vi "6_position_bandwidth_main.vi"() -> ()   [LabVIEW 2019]
uses:
  Shared VIs/ENPID/PID_Settings.ctl
  Shared VIs/ENPID/Gains.ctl
  Shared VIs/ENPID/NonLinearGainParams.ctl
  Shared VIs/ENPID/NonLinearGain.ctl
  Shared VIs/ENPID/DPartVariable.ctl
  Shared VIs/ENPID/VelocityEstimate.ctl
  Shared VIs/ENPID/OutputRange.ctl
  Shared VIs/TypeDef_TDMS_States.ctl
  <vilib>/myRIO/Common/Instrument Driver Framework/myRIO v1.0/Encoder/typedefs/Encoder Signal Mode.ctl
  Shared VIs/ModelSpecific/ETHMikeModel.ctl
  Shared VIs/ModelSpecific/ReadOnlyGlobalActions.ctl
  <vilib>/myRIO/Instrument Drivers/Onboard IO/AO/typedefs/AO Reference.ctl
  <vilib>/myRIO/Common/Instrument Driver Framework/Utilities/typedefs/myRIO Generic Hardware Reference.ctl
  <vilib>/myRIO/Common/Instrument Driver Framework/Utilities/typedefs/Hardware Version Enum.ctl
  <vilib>/myRIO/Common/Instrument Driver Framework/Utilities/typedefs/myRIO v1.0 Reference.ctl
  <vilib>/myRIO/Common/Instrument Driver Framework/Utilities/typedefs/Generic FPGA Reference.ctl
  <vilib>/myRIO/Common/Instrument Driver Framework/myRIO v1.0/AO/typedefs/AO Channels List.ctl
  <vilib>/myRIO/Common/Instrument Driver Framework/myRIO v1.0/AO/typedefs/AO Channels Enum.ctl
  <vilib>/myRIO/Common/Instrument Driver Framework/Utilities/typedefs/Analog Scaling Constants List.ctl
  <vilib>/myRIO/Common/Instrument Driver Framework/Utilities/typedefs/Analog Scaling Constants.ctl
  <vilib>/userDefined/High Color/nirio_resource_hc.ctl
  <vilib>/myRIO/Instrument Drivers/Onboard IO/AI/typedefs/AI Reference.ctl
  <vilib>/myRIO/Common/Instrument Driver Framework/myRIO v1.0/AI/typedefs/AI Channels List.ctl
  <vilib>/myRIO/Common/Instrument Driver Framework/myRIO v1.0/AI/typedefs/AI Channels Enum.ctl
  <vilib>/Platform/TimedLoop/XDataNode/timing_clust.ctl
  <vilib>/Platform/TimedLoop/XDataNode/nitl_modes.ctl
  <vilib>/Platform/TimedLoop/XDataNode/wakeup.ctl
  <vilib>/Analysis/3filter.llb/Filter Passband Type.ctl
  <vilib>/myRIO/Common/Instrument Driver Framework/myRIO v1.0/AO/vis/myRIO v1.1 Open AO.vi
  <vilib>/myRIO/Common/Instrument Driver Framework/myRIO v1.0/AI/vis/myRIO v1.1 Open AI.vi
  <vilib>/myRIO/Common/Instrument Driver Framework/Utilities/vis/Validate Channels.vi
  <vilib>/myRIO/Common/Instrument Driver Framework/myRIO v1.0/AO/vis/myRIO v1.0 Reserve AO.vi
  <vilib>/myRIO/Common/Instrument Driver Framework/myRIO v1.0/AI/vis/myRIO v1.0 Reserve AI.vi
  <vilib>/myRIO/Common/Instrument Driver Framework/myRIO v1.0/AO/vis/myRIO v1.0 Close AO.vi
  <vilib>/myRIO/Common/Instrument Driver Framework/myRIO v1.0/AI/vis/myRIO v1.0 Close AI.vi
  <vilib>/myRIO/Common/Instrument Driver Framework/myRIO v1.0/Encoder/vis/myRIO v1.0 Close Encoder.vi
  <vilib>/myRIO/Common/Instrument Driver Framework/myRIO v1.0/AO/vis/myRIO v1.0 Build MUX Configuration AO.vi
  <vilib>/myRIO/Common/Instrument Driver Framework/myRIO v1.0/Resource Manager/vis/myRIO v1.0 Reserve Channel List.vi
  <vilib>/myRIO/Common/Instrument Driver Framework/myRIO v1.0/AI/vis/myRIO v1.0 Build MUX Configuration AI.vi
  <vilib>/myRIO/Common/Instrument Driver Framework/myRIO v1.0/AO/vis/myRIO v1.0 Unreserve AO.vi
  <vilib>/myRIO/Common/Instrument Driver Framework/myRIO v1.0/AI/vis/myRIO v1.0 Unreserve AI.vi
  <vilib>/myRIO/Common/Instrument Driver Framework/myRIO v1.0/Encoder/vis/myRIO v1.0 Unreserve Encoder.vi
  <vilib>/myRIO/Common/Instrument Driver Framework/myRIO v1.0/Resource Manager/vis/myRIO v1.0 Reserve Channel.vi
  <vilib>/myRIO/Common/Instrument Driver Framework/myRIO v1.0/Resource Manager/vis/myRIO v1.0 Unreserve Channel.vi
  <vilib>/myRIO/Common/Instrument Driver Framework/myRIO v1.0/Resource Manager/vis/myRIO v1.0 Unreserve Channel List.vi
  <vilib>/myRIO/Common/Instrument Driver Framework/myRIO v1.0/Encoder/vis/myRIO v1.0 Build MUX Configuration Encoder.vi
  <vilib>/myRIO/Common/Instrument Driver Framework/myRIO v1.0/Resource Manager/vis/myRIO v1.0 Build Mutex Name.vi
  <vilib>/myRIO/Common/Instrument Driver Framework/myRIO v1.0/Resource Manager/vis/myRIO v1.0 Create Configuration List.vi
  <vilib>/Utility/VariantDataType/GetNumericInfo.vi
  <vilib>/Utility/error.llb/Error Cluster From Error Code.vi
  <vilib>/myRIO/Common/Instrument Driver Framework/myRIO v1.0/myRIO v1.1 Open.vi
  <vilib>/myRIO/Common/Instrument Driver Framework/myRIO v1.0/AO/vis/myRIO v1.0 Get Scaling Constants AO.vi
  <vilib>/myRIO/Common/Instrument Driver Framework/Utilities/vis/IO Manager.vi
  <vilib>/myRIO/Common/Instrument Driver Framework/Utilities/vis/Configuration Manager.vi
  <vilib>/myRIO/Common/Instrument Driver Framework/myRIO v1.0/myRIO v1.0 Close.vi
  <vilib>/myRIO/Common/Instrument Driver Framework/myRIO v1.0/AO/vis/myRIO v1.0 Write AO.vi
  <vilib>/myRIO/Common/Instrument Driver Framework/myRIO v1.0/AI/vis/myRIO v1.0 Get Scaling Constants AI.vi
  <vilib>/myRIO/Common/Instrument Driver Framework/myRIO v1.0/Encoder/vis/myRIO v1.0 Read Encoder.vi
  <vilib>/myRIO/Common/Instrument Driver Framework/myRIO v1.0/AI/vis/myRIO v1.0 Read AI.vi
  <vilib>/myRIO/Common/Instrument Driver Framework/myRIO v1.0/Encoder/vis/myRIO v1.0 Enable Encoder.vi
  <vilib>/myRIO/Common/Instrument Driver Framework/myRIO v1.0/Encoder/vis/myRIO v1.0 Shutdown Encoder.vi
  <vilib>/myRIO/Common/Instrument Driver Framework/myRIO v1.0/Resource Manager/vis/myRIO v1.0 Configure IO.vi
  <vilib>/myRIO/Instrument Drivers/Onboard IO/AO/vis/myRIO AO Open.xnode
  <vilib>/myRIO/Instrument Drivers/Onboard IO/AI/vis/myRIO AI Open.xnode
  <vilib>/platform/TimedLoop/XDataNode/XDataNode.xnode
  <vilib>/myRIO/Instrument Drivers/Onboard IO/AO/AO.lvlib
  <vilib>/myRIO/Instrument Drivers/Onboard IO/Encoder/Encoder.lvlib
  <vilib>/myRIO/Instrument Drivers/Onboard IO/AI/AI.lvlib
  <vilib>/Platform/TimedLoop/XDataNode/XDNodeRunTimeDep.lvlib
  <vilib>/Analysis/NI_AALBase.lvlib
  <vilib>/ptbypt/NI_PtbyPt.lvlib
  <vilib>/addons/control/pid/NI_PID_pid.lvlib
panel:
  out "Velocity [deg/s]":dbl(graph)
  out "TDMS States":T1
  in  "TDMS Storage File Input":string
  in  "PID Settings":T2={"Gains"={"K(e)"=0.0, "Kp"=0.800000011920929, "Ki"=0.0, "Kd"=0.003000000026077032}, "Non-linear gain"={"Non-linear gain P"=enum."off", "Non-linear gain I"=enum."off", "Non-linear gain D"=enum."off"}, "D-Part variable"=enum."process variable", "Velocity estimate dy/dt"=enum."external", "Anti reset windup"=TRUE, "I-Part error band"=inf, "Output range"={"output high"=0.0, "output low"=0.0}}
  in  "Sine Amplitude (deg)":dbl
  out "Current Setpoint [A]":dbl(graph)
  out "i":dbl
  out "Velocity Unfiltered [deg/s]":dbl
  out "Position [deg]":cluster{"Position [deg]":dbl, "setpoint":dbl}(graph)
  out "Time (s)":dbl
  out "Velocity [deg/s]":dbl
  out "Current Setpoint [A]":dbl
  out "Position Setpoint [deg]":dbl
  in  "Sine Frequency (Hz)":dbl
  in  "Cycles":dbl
  in  "run":bool
  in  "Save data?":bool
  out "Position [deg]":dbl
  in  "stop":bool
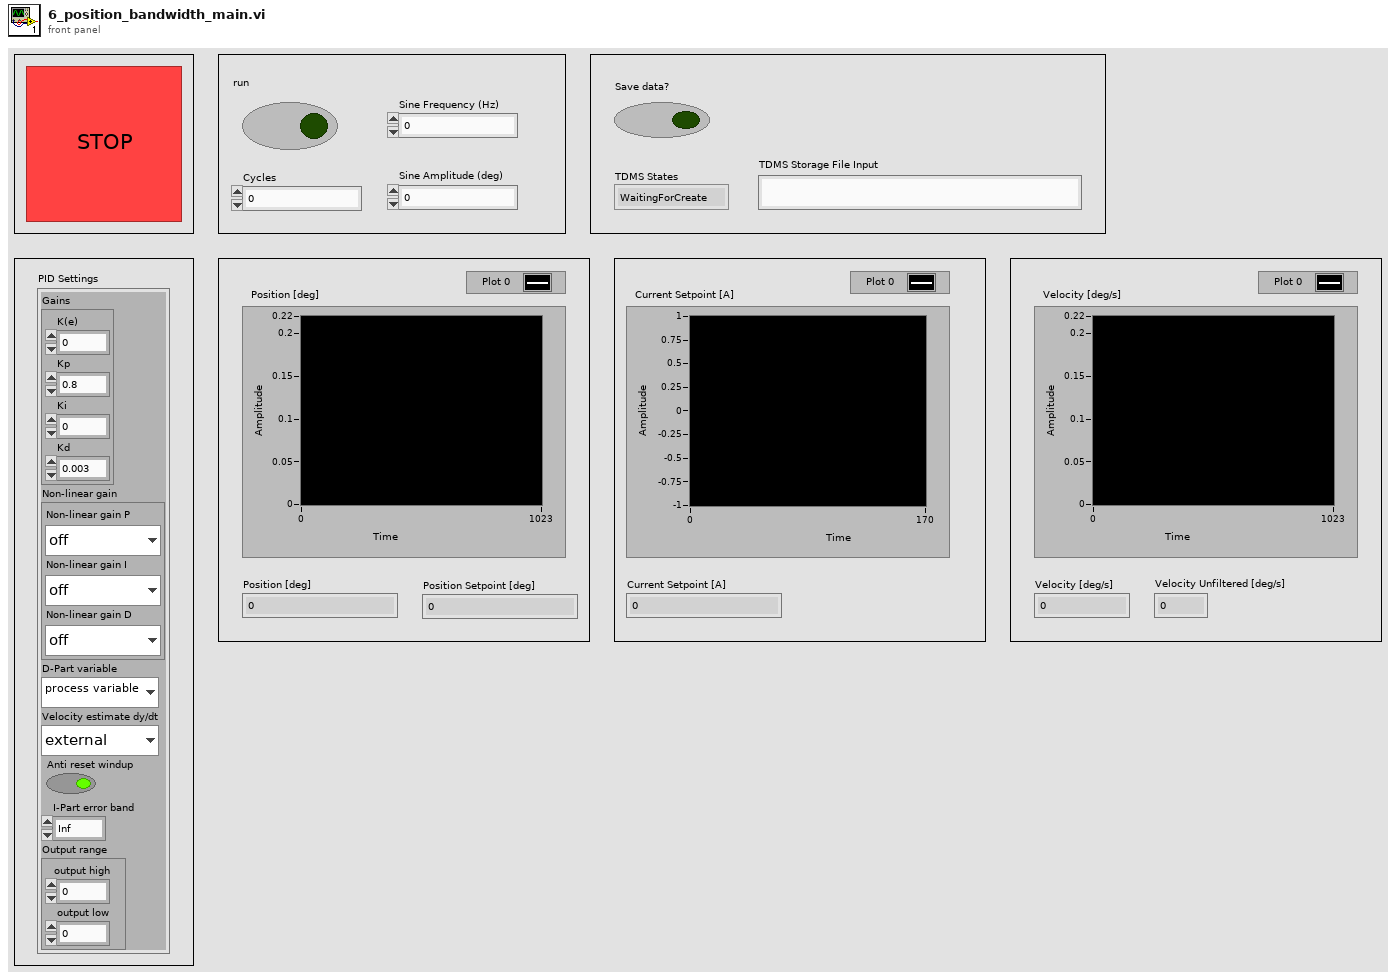
[diagram p1: front panel]
types:
  T1 = typedef "TypeDef_TDMS_States.ctl" = enum16{"WaitingForCreate", "Create", "Buffering", "Flushing", "Write", "Close"}
  T2 = typedef "PID_Settings.ctl" = cluster{"Gains":T3, "Non-linear gain":T4, "D-Part variable":T6, "Velocity estimate dy/dt":T7, "Anti reset windup":bool, "I-Part error band":dbl, "Output range":T8}
  T3 = typedef "Gains.ctl" = cluster{"K(e)":dbl, "Kp":dbl, "Ki":dbl, "Kd":dbl}
  T4 = typedef "NonLinearGainParams.ctl" = cluster{"Non-linear gain P":T5, "Non-linear gain I":T5, "Non-linear gain D":T5}
  T5 = typedef "NonLinearGain.ctl" = enum16{"exponential", "quadratic", "off"}
  T6 = typedef "DPartVariable.ctl" = enum16{"error", "process variable"}
  T7 = typedef "VelocityEstimate.ctl" = enum16{"derivative", "external"}
  T8 = typedef "OutputRange.ctl" = cluster{"output high":dbl, "output low":dbl}
  T9 = typedef "nirio_resource_hc.ctl" = tag
  T10 = typedef "Hardware Version Enum.ctl" = enum16{"Unknown", "myRIO-1900", "myRIO-1950", "roboRIO", "NI ELVIS RIO CM", "ELVIS III"}
  T11 = enum16{"open", "open or create", "create or replace", "create", "open (read-only)"}
  T12 = typedef "XDNodeRunTimeDep.lvlib/timing_clust.ctl" = cluster{"Expected End [f-1]":u64, "Actual End [f-1]":u64, "Finished Late? [f-1]":bool, "Expected End [i-1]":u64, "Actual End [i-1]":u64, "Finished Late? [i-1]":bool, "Expected Start [i]":u64, "Actual Start [i]":u64, "Expected Start [f]":u64, "Actual Start [f]":u64, "Source Name":string, "Structure Name":string, "Period":i64, "Deadline":i64, "Offset":i64, "Start":i64, "Priority":i32, "Timeout":i32, "Mode":T13, "Wakeup Reason":T14, "Error":errorcluster, "Source Type":string, "Secondary Source Type":string, "Global End Time":u64, "Global Start Time":u64, "Frame Duration":u64, "Iteration Duration":u64, "Assigned CPU":i32, "I/O Scan Engine Mode":u32}
  T13 = typedef "XDNodeRunTimeDep.lvlib/nitl_modes.ctl" = enum32{"No Change", "Process missed periods, maintain original phase", "Discard missed periods, maintain original phase", "Process missed periods, ignore original phase", "Discard missed periods, ignore original phase"}
  T14 = typedef "XDNodeRunTimeDep.lvlib/wakeup.ctl" = enum32{"Normal", "Aborted", "Asynchronous wakeup", "Timing source error", "Timed loop error", "Timeout"}
  T15 = typedef "NI_AALBase.lvlib/Filter Passband Type.ctl" = enum32{"Lowpass", "Highpass", "Bandpass", "Bandstop"}
  T16 = typedef "ReadOnlyGlobalActions.ctl" = enum16{"Initialize", "Read", "Write"}
  T17 = typedef "ETHMikeModel.ctl" = enum16{"ETH Mike #1", "ETH Mike #2", "ETH Mike #3", "ETH Mike #4", "ETH MIKE #5"}
  T18 = typedef "Encoder Signal Mode.ctl" = enum16{"Quadrature phase signal", "Step and direction signal"}
  T19 = typedef "AO.lvlib/AO Reference.ctl" = cluster{"myRIO Reference":T20, "AO Channel List":T23, "AO Scaling Constant List":T25}
  T20 = typedef "myRIO Generic Hardware Reference.ctl" = cluster{"myRIO Model":T10, "myRIO Hardware Reference":T21}
  T21 = typedef "myRIO v1.0 Reference.ctl" = cluster{"Generic FPGA Reference":T22, "Allow multiple opens":bool}
  T22 = typedef "Generic FPGA Reference.ctl" = refnum<k20>
  T23 = typedef "AO Channels List.ctl" = T24[]
  T24 = typedef "AO Channels Enum.ctl" = enum16{"Not Connected", "AudioOut/Left", "AudioOut/Right", "C/AO0", "C/AO1", "A/AO0", "A/AO1", "B/AO0", "B/AO1"}
  T25 = typedef "Analog Scaling Constants List.ctl" = T26[]
  T26 = typedef "Analog Scaling Constants.ctl" = cluster{"LSB Weight (Volts)":dbl, "Offset (Volts)":dbl, "Signed?":bool}
  T27 = typedef "Encoder.lvlib/Encoder Reference.ctl" = cluster{"myRIO Reference":T20, "Encoder Channels Enum":T28}
  T28 = typedef "Encoder Channels Enum.ctl" = enum16{"Not Connected", "C/ENC0", "C/ENC1", "A/ENC", "A/ENC0", "A/ENC1", "A/ENC2", "A/ENC3", "A/ENC4", "A/ENC5", "A/ENC6", "A/ENC7", "A/ENC8", "A/ENC9", "B/ENC", "B/ENC0", "B/ENC1", "B/ENC2", "B/ENC3", "B/ENC4", "B/ENC5", "B/ENC6", "B/ENC7", "B/ENC8", "B/ENC9", "DIO/ENC0", "DIO/ENC1", "DIO/ENC2", "DIO/ENC3", "DIO/ENC4"}
  T29 = typedef "AI.lvlib/AI Reference.ctl" = cluster{"myRIO Reference":T20, "AI Channels List":T30, "AI Scaling Constants List":T25}
  T30 = typedef "AI Channels List.ctl" = T31[]
  T31 = typedef "AI Channels Enum.ctl" = enum16{"Not Connected", "AudioIn/Left", "AudioIn/Right", "C/AI0", "C/AI1", "A/AI0", "A/AI1", "A/AI2", "A/AI3", "A/AI4", "A/AI5", "A/AI6", "A/AI7", "B/AI0", "B/AI1", "B/AI2", "B/AI3", "B/AI4", "B/AI5", "B/AI6", "B/AI7", "AI/AI0", "AI/AI1", "AI/AI2", "AI/AI3", "A/AI0 (DIFF)", "A/AI1 (DIFF)", "A/AI2 (DIFF)", "A/AI3 (DIFF)", "B/AI0 (DIFF)", "B/AI1 (DIFF)", "B/AI2 (DIFF)", "B/AI3 (DIFF)"}
  T32 = typedef "TypeDefTachometerParam.ctl" = cluster{"Offset [V]":dbl, "Gain [deg/sV]":dbl}
  T33 = cluster{"Position [deg]":dbl, "Position [deg]":dbl}
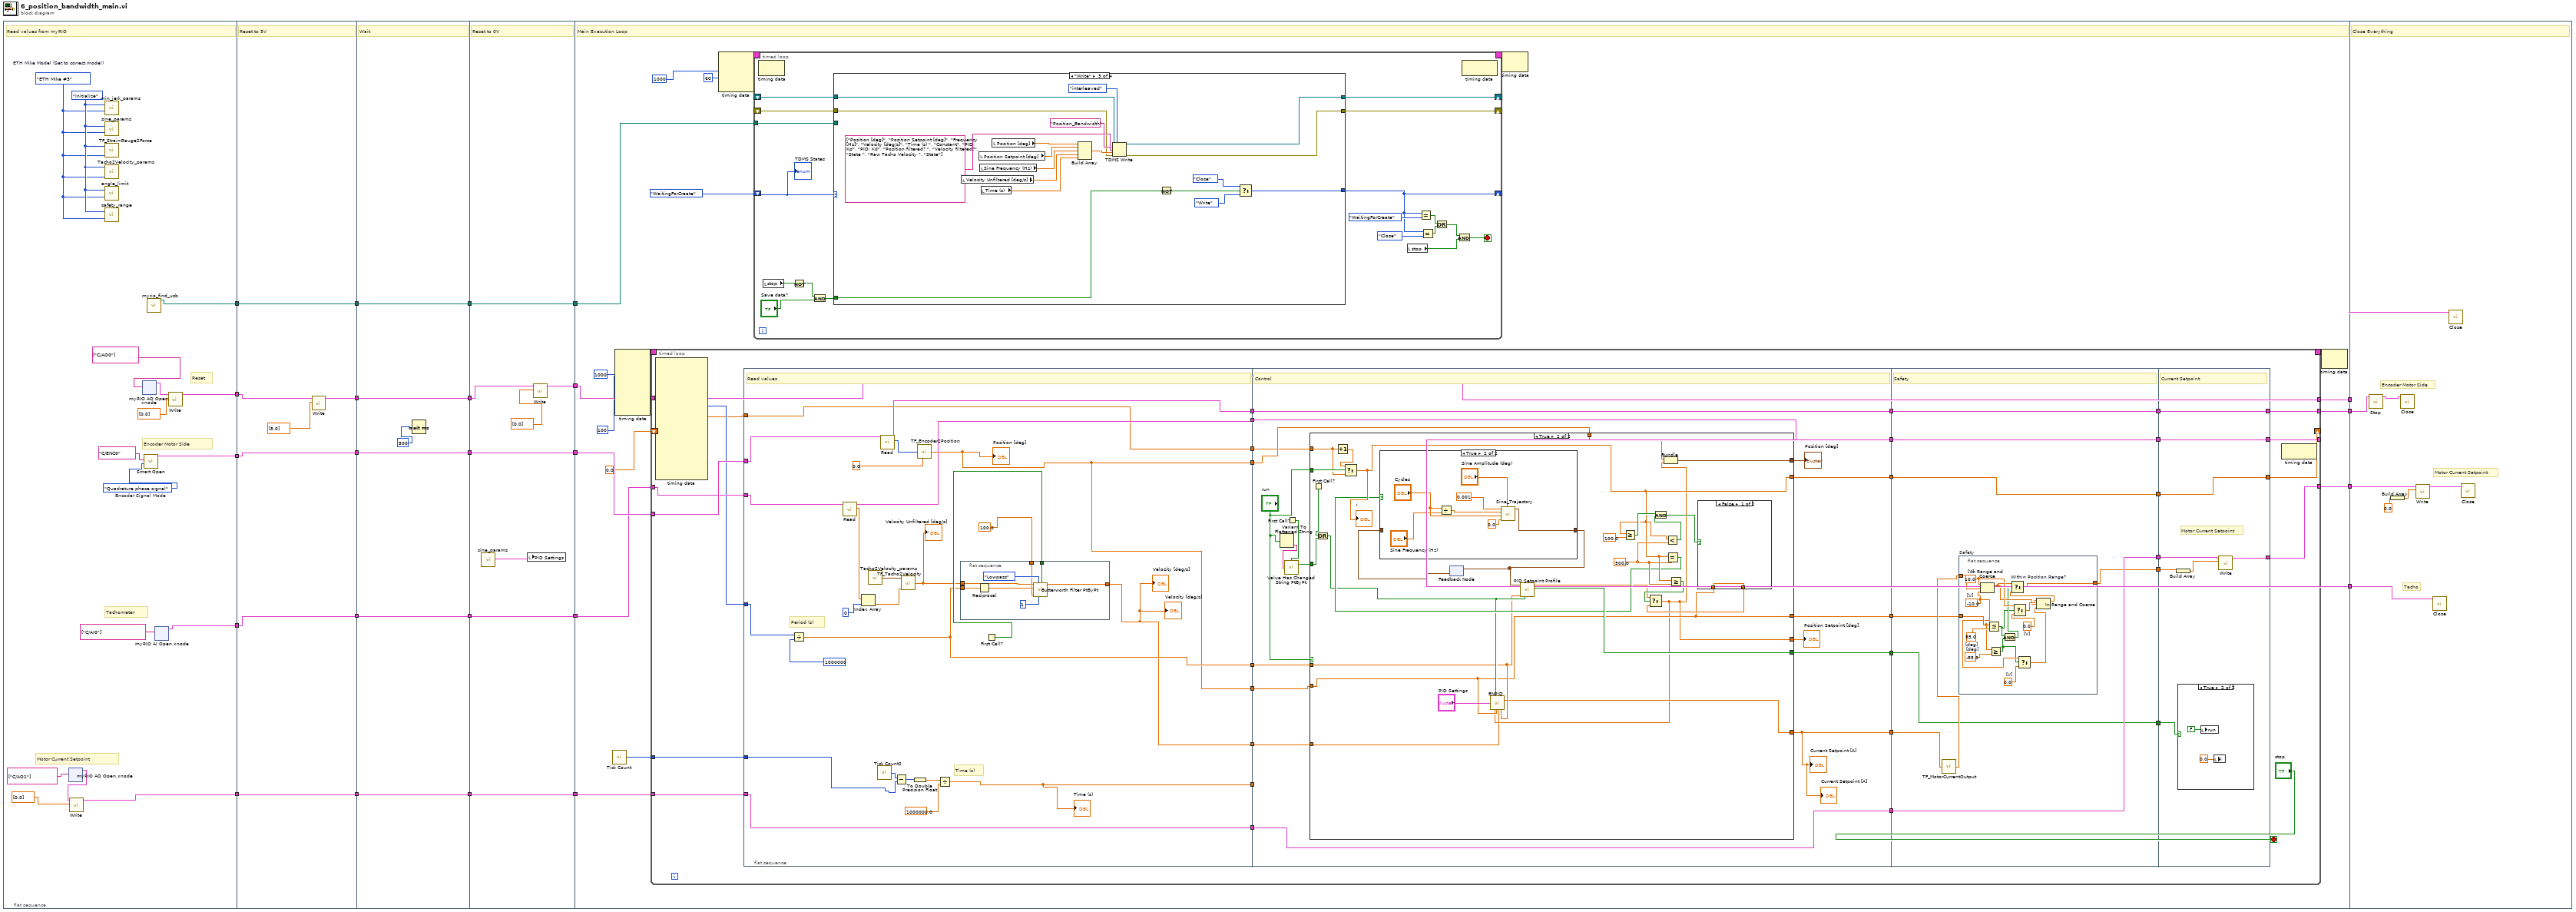
[diagram p0: block diagram]
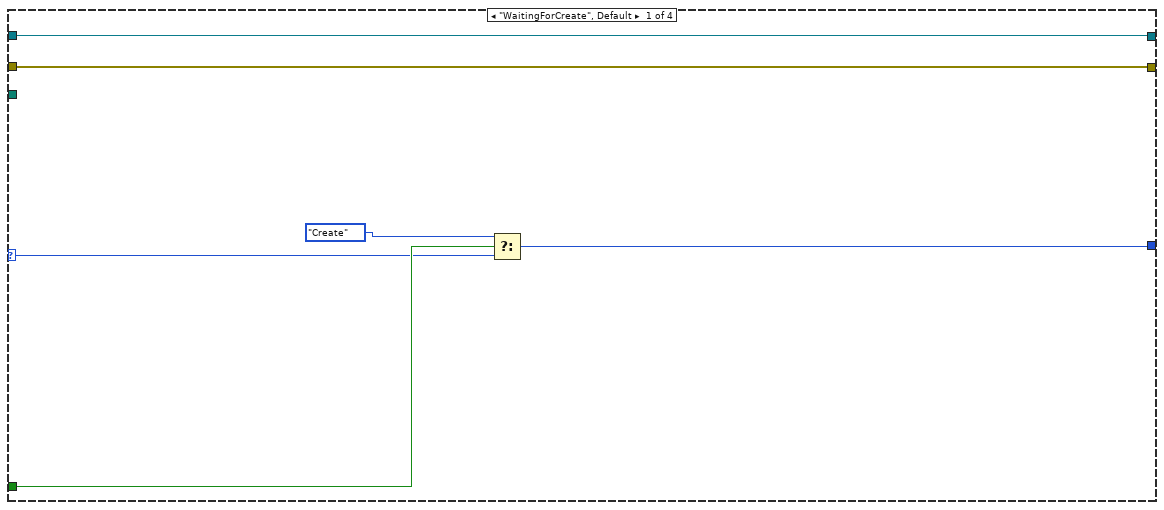
[diagram p2: hidden frame]
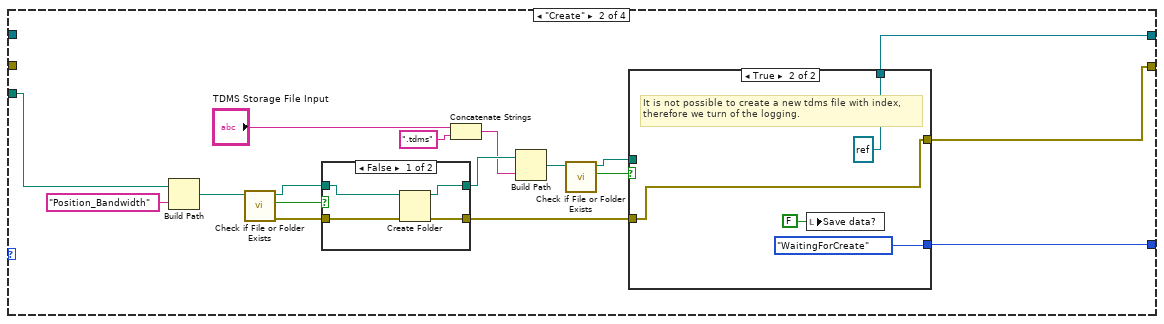
[diagram p3: hidden frame]
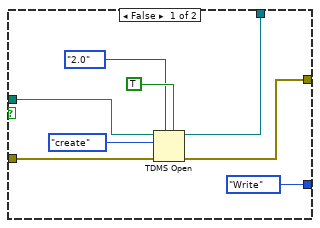
[diagram p4: hidden frame]
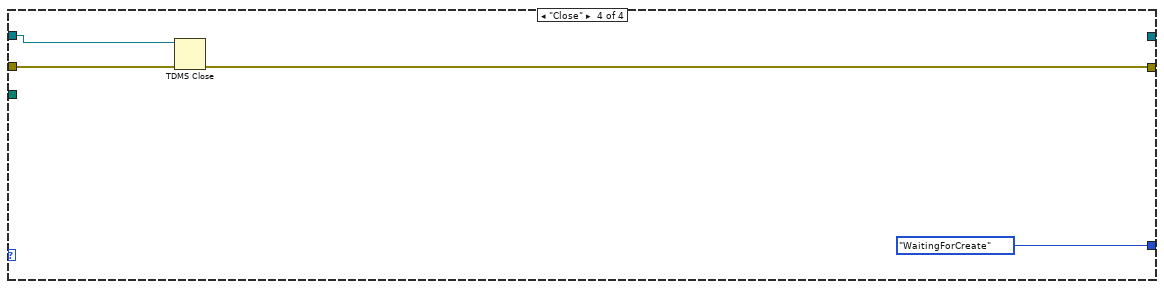
[diagram p6: hidden frame]
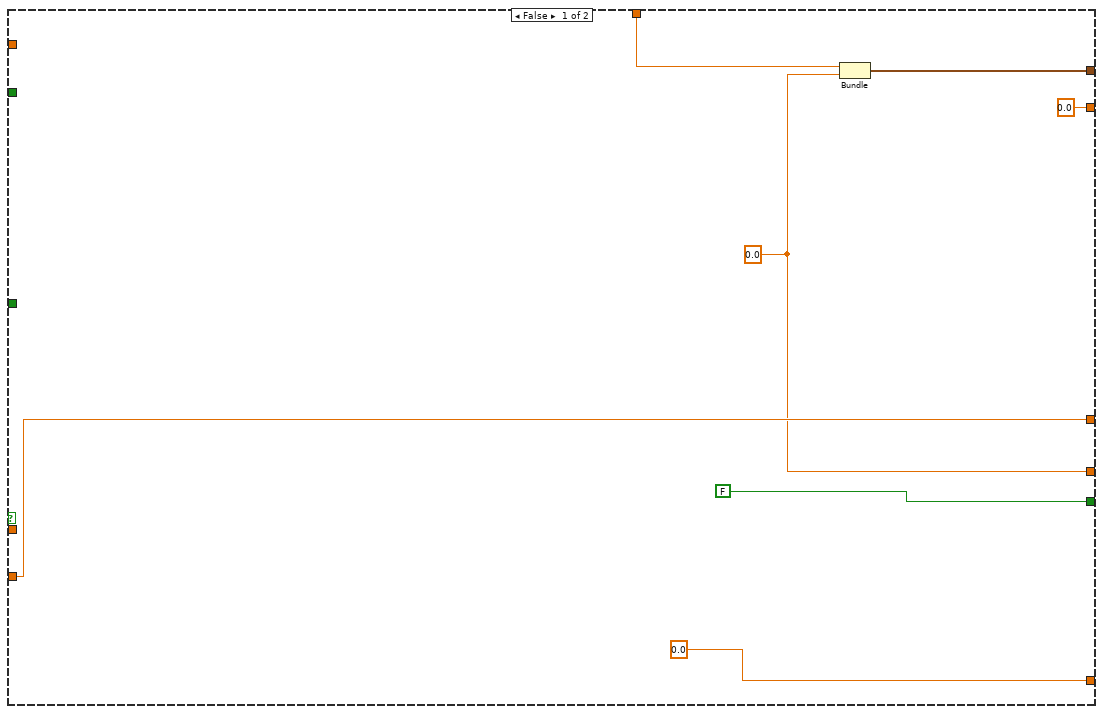
[diagram p7: hidden frame]
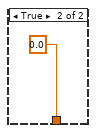
[diagram p8: hidden frame]
diagram:
  n1 = flat-sequence {
    tunnel: [w34] -> w24
    tunnel: [w33] -> w23
    tunnel: [w32] -> w22
    tunnel: [w31] -> w21
    tunnel: [w27] -> w2
    tunnel: w24 -> [w96]
    tunnel: w23 -> [w100]
    tunnel: w22 -> [w98]
    tunnel: w21 -> [w97]
    tunnel: [w99] -> w20
    tunnel: [w98] -> w15
    tunnel: [w97] -> w12
    tunnel: [w96] -> w6
    tunnel: [w95] -> w3
    tunnel: w2 -> [w95]
    tunnel: w20 -> [w106]
    tunnel: [w106] -> w19
    tunnel: [w105] -> w16
    tunnel: w15 -> [w105]
    tunnel: [w104] -> w13
    tunnel: w12 -> [w104]
    tunnel: [w103] -> w7
    tunnel: w6 -> [w103]
    tunnel: [w102] -> w4
    tunnel: w3 -> [w102]
    tunnel: w19 -> [w114]
    tunnel: [w113] -> w18
    tunnel: [w112] -> w17
    tunnel: w16 -> [w112]
    tunnel: [w111] -> w14
    tunnel: w13 -> [w111]
    tunnel: [w110] -> w8
    tunnel: w7 -> [w110]
    tunnel: [w109] -> w5
    tunnel: w4 -> [w109]
    tunnel: w18 -> [w132]
    tunnel: w17 -> [w131]
    tunnel: w14 -> [w129]
    tunnel: [w120] -> w11
    tunnel: [w130] -> w10
    tunnel: [w128] -> w9
    tunnel: w8 -> [w125]
    tunnel: w5 -> [w122]
    tunnel: [w121] -> w1
    tunnel: w11 -> [w404]
    tunnel: w10 -> [w402]
    tunnel: w9 -> [w401]
    tunnel: w1 -> [w399]
    frame #0 {
      w26 = ReadOnlyGlobalActions."Initialize" ("Action (Read)")
      w25 = ETHMikeModel."ETH Mike #3"  # ETH Mike Model (Set to correct model)
      w36 = Encoder_Signal_Mode."Quadrature phase signal"  # Encoder Signal Mode
      # "Motor Current Setpoint"
      # "Tachometer"
      # "Encoder Motor Side"
      # "Reset"
      # "Read values from myRIO"
      n2 = xnode "myRIO AO Open.xnode"("Channel Names"=tag[] ["C/AO1"]) -> ("AO Ref Out"=w29:T19)  [unwired: 2 in, 1 out]
      n3 = call <vilib>:"Write.vi"("Values"=dbl[] [0.0], "AO Ref In"=w29) -> ("AO Ref Out"=w27:T19)  [unwired: 7 in, 1 out]
      n4 = call "min_jerk_params.vi"("Action (Read)"=w26, "ETH Mike Model"=w25) -> ()  [unwired: 17 in, 1 out]
      n5 = call "sine_params.vi"("Action (Read)"=w26, "ETH Mike Model"=w25) -> ()  [unwired: 17 in, 1 out]
      n6 = call "TF_StrainGauge2Force.vi"("Action (Read)"=w26, "ETH Mike Model"=w25) -> ()  [unwired: 3 in, 1 out]
      n7 = call "Tacho2Velocity_params.vi"("Action (Read)"=w26, "ETH Mike Model"=w25) -> ()  [unwired: 3 in, 1 out]
      n8 = call "angle_limit.vi"("ETH Mike Model"=w25, "Action (Read)"=w26) -> ()  [unwired: 1 out]
      n9 = call "safety_range.vi"("ETH Mike Model"=w25, "Action (Read)"=w26) -> ()  [unwired: 1 out]
      n10 = xnode "myRIO AO Open.xnode"("Channel Names"=tag[] ["C/AO0"]) -> ("AO Ref Out"=w39:T19)  [unwired: 2 in, 1 out]
      n11 = call <vilib>:"Smart Open.vi"("Encoder Signal Mode"=w36, "Channel Name"=tag "C/ENC0") -> ("Encoder Ref Out"=w32:T27)  [unwired: 8 in, 1 out]
      n12 = call "myrio_find_usb.vi"() -> ("Largest USB Partition Path"=w34:path)  [unwired: 9 in, 2 out]
      n13 = xnode "myRIO AI Open.xnode"("Channel Names"=tag[] ["C/AI0"]) -> ("AI Ref Out"=w31:T29)  [unwired: 2 in, 1 out]
      n14 = call <vilib>:"Write.vi"("Values"=dbl[] [0.0], "AO Ref In"=w39) -> ("AO Ref Out"=w33:T19)  [unwired: 7 in, 1 out]
    }
    frame #1 {
      # "Reset to 5V"
      n15 = call <vilib>:"Write.vi"("Values"=dbl[] [5.0], "AO Ref In"=w100) -> ("AO Ref Out"=w99:T19)  [unwired: 7 in, 1 out]
    }
    frame #2 {
      # "Wait"
      n16 = Wait (ms)(milliseconds to wait=500) -> ()  [unwired: 1 out]
    }
    frame #3 {
      # "Reset to 0V"
      n17 = call "sine_params.vi"() -> ("PID Settings"=w108:T2)  [unwired: 19 in]
      n18 = local write "PID Settings"(w108) -> ()
      n19 = call <vilib>:"Write.vi"("Values"=dbl[] [0.0], "AO Ref In"=w114) -> ("AO Ref Out"=w113:T19)  [unwired: 7 in, 1 out]
    }
    frame #4 {
      # "Main Execution Loop"
      n20 = call "Tick Count"() -> ("Tick Count(uSec)"=w123:u32)
      n21 = node-c288(i64 1000 ("Period"), 100) -> (w135:T12)  [unwired: 6 in]
      n22 = timed-loop {
        timing: w135 -> [_]
        timing-out: [_] -> w134
        tunnel: [w257] -> w120
        tunnel: w132 -> [w257]
        tunnel: w131 -> [w256]
        tunnel: [w255] -> w130
        tunnel: w129 -> [w254]
        tunnel: [w253] -> w128
        tunnel: w123 -> [w244]
        tunnel: w122 -> [w237]
        tunnel: [w233] -> w121
        shift-right: [w227] -> _
        shift-left: 0.0 -> [w224]
        stop <- "stop" stop-if-true
        n23 = node-c288() -> (w252:i64)  [unwired: 1 in, 16 out]
        n24 = flat-sequence {
          tunnel: [w283] -> w251
          tunnel: [w273] -> w249
          tunnel: w252 -> [w281]
          tunnel: w254 -> [w282]
          tunnel: w256 -> [w274]
          tunnel: w244 -> [w268]
          tunnel: [w265] -> w243
          tunnel: [w267] -> w242
          tunnel: [w258] -> w241
          tunnel: [w264] -> w240
          tunnel: w237 -> [w266]
          tunnel: [w266] -> w236
          tunnel: [w264] -> w230
          tunnel: [w262] -> w228
          tunnel: w224 -> [w262]
          tunnel: w251 -> [w309]
          tunnel: [w309] -> w250
          tunnel: w249 -> [w308]
          tunnel: [w308] -> w248
          tunnel: w243 -> [_]
          tunnel: w242 -> [w307]
          tunnel: w241 -> [w303]
          tunnel: w240 -> [w302]
          tunnel: [w301] -> w239
          tunnel: w236 -> [w300]
          tunnel: [w300] -> w235
          tunnel: [w299] -> w231
          tunnel: w230 -> [w298]
          tunnel: [w294] -> w229
          tunnel: w228 -> [w297]
          tunnel: [w295] -> w225
          tunnel: w250 -> [w362]
          tunnel: w248 -> [w361]
          tunnel: [w362] -> w246
          tunnel: [w361] -> w245
          tunnel: w239 -> [w359]
          tunnel: [w354] -> w238
          tunnel: w235 -> [w358]
          tunnel: [w358] -> w234
          tunnel: [w357] -> w232
          tunnel: w231 -> [w357]
          tunnel: w229 -> [w356]
          tunnel: [w355] -> w226
          tunnel: w225 -> [w355]
          tunnel: [w385] -> w253
          tunnel: [w386] -> w255
          tunnel: w246 -> [w386]
          tunnel: w245 -> [w385]
          tunnel: w238 -> [w384]
          tunnel: [w382] -> w233
          tunnel: w234 -> [w381]
          tunnel: w232 -> [w380]
          tunnel: [w379] -> w227
          tunnel: w226 -> [w379]
          frame #0 {
            # "Time (s)"
            # "Period (s)"
            # "Read values"
            n25 = Divide(x=w281, y=1000000) -> (x/y=w267:dbl)
            n26 = call <vilib>:"Read.vi"("AI Ref In"=w282) -> ("Values"=w278:dbl[], "AI Ref Out"=w273:T29)  [unwired: 8 in, 1 out]
            n27 = Index Array(array=w278, index=0) -> (element=w260:dbl)
            n28 = call "Tacho2Velocity_params.vi"() -> ("Cluster"=w261:T32)  [unwired: 5 in]
            n29 = call "Tick Count2"() -> ("Tick Count(uSec)"=w272:u32)
            n30 = call <vilib>:"Read.vi"("Encoder Ref In"=w274) -> ("Counter Value"=w280:i32, "Encoder Ref Out"=w283:T27)  [unwired: 6 in, 3 out]
            n31 = Subtract(x=w272, y=w268) -> (x-y=w271:u32)
            n32 = call "TF_Tacho2Velocity.vi"("Tachometer Voltage [V]"=w260, "Tachometer param"=w261) -> ("Tachometer Velocity [deg/s]"=w259:dbl)  [unwired: 2 in]
            "Velocity Unfiltered [deg/s]" <- w259
            n33 = To Double Precision Float(number=w271) -> (double precision float=w270:dbl)
            n34 = call "TF_Encoder2Position.vi"("Counter Value"=w280, "Offset"=0.0) -> ("Position [deg]"=w264:dbl)  [unwired: 3 in]
            "Position [deg]" <- w264
            n35 = Divide(x=w270, y=1000000.0) -> (x/y=w265:dbl)
            "Time (s)" <- w265
            n36 = flat-sequence {
              tunnel: w259 -> [w291]
              tunnel: w267 -> [w289]
              tunnel: [w286] -> w258
              tunnel: w275 -> [w285]
              tunnel: 100.0 -> [w284]
              frame #0 {
                n37 = Reciprocal(x=w289) -> (1/x=w290:dbl)
                n38 = call <vilib>:"Butterworth Filter PtByPt.vi"("initialize"=w285, "order"=1, "filter type"=Filter_Passband_Type."Lowpass", "low cutoff freq: fl"=w284, "sampling freq: fs"=w290, "x"=w291) -> ("Filtered x"=w286:dbl)  [unwired: 3 in, 1 out]
              }
            }
            n39 = First Call?() -> (First Call?: T/F=w275:bool)
            "Velocity [deg/s]" <- w258
            "Velocity [deg/s]" <- w258
          }
          frame #1 {
            # "Control"
            n40 = Variant To Flattened String(Variant="run") -> (data string=w306:string)  [unwired: 1 out]
            n41 = First Call?() -> (First Call?: T/F=w305:bool)
            n42 = call "Value Has Changed String PtByPt.vi"("input data point"=w306, "initialize"=w305) -> ("has changed"=w304:bool)  [unwired: 1 out]
            n43 = case shown="True" "run" {
              tunnel: w302 -> [w315 w319]
              tunnel: w307 -> [_ w321]
              tunnel: w304 -> [_ w343]
              tunnel: w303 -> [_ w322]
              tunnel: [0.0 w320] -> w294
              tunnel: [w315 w319] -> w301
              tunnel: [FALSE ("profile complete?") w341] -> w299
              tunnel: w298 -> [w312 w330]
              tunnel: w297 -> [_ w336]
              tunnel: "run" -> [_ w338]
              tunnel: [0.0 w329] -> w295
              tunnel: [w310 w318] -> w293
              tunnel: [w311 w317] -> w292
              frame False {
                w310 = 0.0
                n44 = Bundle("Position [deg]"=w312, w310) -> (w311:cluster{"Position [deg]":dbl, dbl})  [unwired: 1 in]
              }
              frame True {
                w328 = 500.0 ("y")
                n45 = First Call?() -> (First Call?: T/F=w342:bool)
                n46 = Or(x=w342, y=w343) -> (x .or. y?=w325:bool)
                n47 = Increment(x=w336) -> (x+1=w337:dbl)
                n48 = Select(t=w337, s=w338, f=w336) -> (s? t:f=w329:dbl)
                "i" <- w329
                n49 = feedback #1() -> (w339:cluster{"time (s)":dbl, "setpoint":dbl}[])  [unwired: 1 in]
                n50 = Greater Or Equal?(x=w329, y=100.0) -> (x >= y?=w332:bool)
                n51 = Less?(x=w329, y=w328) -> (x < y?=w333:bool)
                n52 = And(x=w332, y=w333) -> (x .and. y?=w331:bool)
                n53 = Equal?(x=w329, y=w328) -> (x = y?=w326:bool)
                n54 = case shown="True" w326 {
                  tunnel: [w346 w352] -> w340
                  tunnel: w339 -> [w346 _]
                  frame False {
                  }
                  frame True {
                    n55 = Divide(x="Cycles", y="Sine Frequency (Hz)") -> (x/y=w347:dbl)
                    n56 = call "Sine_Trajectory.vi"("Amplitude"="Sine Amplitude (deg)", "Middle Position"=0.0 ("Offset"), "Cycles"="Cycles", "Duration (s)"=w347, "Sampling Period (s)"=0.001) -> ("Profile"=w352:cluster{"time (s)":dbl, "setpoint":dbl}[])  [unwired: 6 in]
                  }
                }
                n57 = feedback-in #1(w340) -> ()
                n58 = call <vilib>:"PID Setpoint Profile.vi"("reinitialize? (F)"=w325, "dt (s)"=w321, "setpoint profile"=w340) -> ("profile complete?"=w341:bool, "setpoint"=w323:dbl)  [unwired: 3 in, 2 out]
                n59 = Greater Or Equal?(x=w329, y=w328) -> (x >= y?=w327:bool)
                n60 = case shown="False" w331 {
                  tunnel: [w344 0.0] -> w334
                  tunnel: w319 -> [w344 _]
                  frame False {
                  }
                  frame True {
                  }
                }
                n61 = Select(t=w323, s=w327, f=w334) -> (s? t:f=w318:dbl)
                n62 = call "ENPID.vi"("PID Settings"="PID Settings", "r"=w318, "Reset?"=w325, "y"=w319, "dy/dt"=w322, "dt (s)"=w321) -> ("u"=w320:dbl)  [unwired: 12 in, 1 out]
                n63 = Bundle("Position [deg]"=w330, "Position [deg]"=w318) -> (w317:T33)  [unwired: 1 in]
              }
            }
            "Current Setpoint [A]" <- w294
            "Current Setpoint [A]" <- w294
            "Position Setpoint [deg]" <- w293
            "Position [deg]" <- w292
          }
          frame #2 {
            # "Safety"
            n64 = call "TF_MotorCurrentOutput.vi"("Motor Current Setpoint [A]"=w356) -> ("Motor Current Setpoint [V]"=w360:dbl)
            n65 = flat-sequence "Safety" {
              tunnel: w360 -> [w378]
              tunnel: [w377] -> w354
              tunnel: w359 -> [w374]
              frame #0 {
                w366 = 0.0  # [V]
                w372 = 0.0  # [V]
                w375 = -85.0  # [deg]
                w376 = 85.0  # [deg]
                w368 = -10.0  # [V]
                w373 = 10.0  # [V]
                n66 = In Range and Coerce(upper limit=w373, x=w378, lower limit=w368) -> (coerced(x)=w369:dbl)  [unwired: 1 out]
                n67 = Less Or Equal?(x=w374, y=w376) -> (x <= y?=w363:bool)
                n68 = Greater Or Equal?(x=w374, y=w375) -> (x >= y?=w367:bool)
                n69 = And(x=w363, y=w367) -> (x .and. y?=w364:bool)
                n70 = Select(t=w373, s=w363, f=w372) -> (s? t:f=w370:dbl)
                n71 = Select(t=w368, s=w367, f=w366) -> (s? t:f=w365:dbl)
                n72 = In Range and Coerce(upper limit=w370, x=w369, lower limit=w365) -> (coerced(x)=w371:dbl)  [unwired: 1 out]
                n73 = Select "Within Position Range?"(t=w369, s=w364, f=w371) -> (s? t:f=w377:dbl)
              }
            }
          }
          frame #3 {
            # "Motor Current Setpoint"
            # "Current Setpoint"
            n74 = Build Array(w384) -> (w383:dbl[])
            n75 = case shown="True" w380 {
              frame False {
              }
              frame True {
                n76 = local write "run"(FALSE ("run")) -> ()
                n77 = local write "i"(0.0 ("i")) -> ()
              }
            }
            n78 = call <vilib>:"Write.vi"("Values"=w383, "AO Ref In"=w381) -> ("AO Ref Out"=w382:T19)  [unwired: 7 in, 1 out]
          }
        }
        n79 = node-c288() -> ()  [unwired: 1 in, 1 out]
      }
      n80 = node-c288(i64 1000 ("Period"), 60 ("Priority")) -> (w127:T12)  [unwired: 2 in]
      n81 = timed-loop {
        timing: w127 -> [_]
        timing-out: [_] -> w126
        shift-right: [w153] -> _
        shift-left: _ -> [w151]
        shift-right: [w152] -> _
        shift-left: _ -> [w150]
        tunnel: w125 -> [w149]
        shift-right: [w139] -> _
        shift-left: TypeDef_TDMS_States."WaitingForCreate" ("TDMS States") -> [w136]
        stop <- w138 stop-if-true
        n82 = node-c288() -> ()  [unwired: 1 in, 1 out]
        n83 = local read "stop"() -> (w145:bool)
        n84 = Not(x=w145) -> (.not. x?=w148:bool)
        n85 = And(x=w148, y="Save data?") -> (x .and. y?=w147:bool)
        n86 = case shown="\"Write\"" w136 {
          selector: w136 -> [w157 _ _ _]
          tunnel: w147 -> [w158 _ w202 _]
          tunnel: [w155 w161 w200 w214] -> w152
          tunnel: [w154 w160 w199 _] -> w153
          tunnel: w151 -> [w154 _ w207 w215]
          tunnel: w150 -> [w155 _ w208 w216]
          tunnel: w149 -> [_ w166 _ _]
          tunnel: [w156 w164 w201 TypeDef_TDMS_States."WaitingForCreate" ("TDMS States")] -> w139
          frame "WaitingForCreate", Default {
            n87 = Select(t=TypeDef_TDMS_States."Create" ("TDMS States"), s=w158, f=w157) -> (s? t:f=w156:T1)
          }
          frame "Create" {
            n88 = Build Path(base path=w166, name or relative path="Position_Bandwidth") -> (appended path=w168:path)
            n89 = call <vilib>:"Check if File or Folder Exists.vi"("path"=w168) -> ("error out"=w174:errorcluster, "file or folder exists?"=w176:bool, "dup path"=w175:path)  [unwired: 8 in]
            n90 = case shown="False" w176 {
              tunnel: w175 -> [w192 w193]
              tunnel: [w191 w194] -> w163
              tunnel: w174 -> [w190 w194]
              tunnel: [w189 w193] -> w173
              frame False {
                n91 = Create Folder(path (use dialog)=w192, error in=w190) -> (created path=w189:path, error out=w191:errorcluster)  [unwired: 1 in, 1 out]
              }
              frame True {
              }
            }
            n92 = Concatenate Strings("TDMS Storage File Input", ".tdms") -> (w170:string)
            n93 = Build Path(base path=w173, name or relative path=w170) -> (appended path=w169:path)
            n94 = call <vilib>:"Check if File or Folder Exists.vi"("path"=w169) -> ("file or folder exists?"=w165:bool, "dup path"=w162:path)  [unwired: 8 in, 1 out]
            n95 = case shown="True" w165 {
              tunnel: [TypeDef_TDMS_States."Write" ("TDMS States") TypeDef_TDMS_States."WaitingForCreate" ("TDMS States")] -> w164
              tunnel: w163 -> [w180 w185]
              tunnel: w162 -> [w179 _]
              tunnel: [w178 w185] -> w161
              tunnel: [w177 refnum<k34> refnum ("tdms file out")] -> w160
              frame False {
                n96 = TDMS Open(5:TRUE, 7:enum16{"1.0", "2.0"}."2.0" ("file format version (2.0)"), 8:w180, 10:T11."create" ("operation (0:open)"), 11:w179) -> (0:w178:errorcluster, 3:w177:refnum<k34>)  [unwired: 2 in]
              }
              frame True {
                # "It is not possible to create a new tdms file with index,\ntherefore we turn of the logging."
                n97 = local write "Save data?"(FALSE ("Save data?")) -> ()
              }
            }
          }
          frame "Write" {
            n98 = local read "Velocity Unfiltered [deg/s]"() -> (w196:dbl)
            n99 = local read "Position Setpoint [deg]"() -> (w198:dbl)
            n100 = local read "Sine Frequency (Hz)"() -> (w197:dbl)
            n101 = local read "Time (s)"() -> (w195:dbl)
            n102 = local read "Position [deg]"() -> (w212:dbl)
            n103 = Build Array(w212, w198, w197, w196, w195) -> (w211:dbl[])
            n104 = TDMS Write(0:w207, 1:enum16{"decimated", "interleaved"}."interleaved" ("data layout (0:decimated)"), 5:"Position_Bandwidth" ("group name in (Untitled)"), 7:string[] ["Position [deg]", "Position Setpoint [deg]", "Frequency [Hz]", "Velocity [deg/s]", "Time (s) ", "Constant", "PID: Kp", "PID: Kd", "Position filtered? ", "Velocity filtered?", "State ", "Raw Tacho Velocity ", "State"], 9:w211, 11:w208) -> (4:w199:refnum<k34>, 15:w200:errorcluster)  [unwired: 2 out]
            n105 = Not(x=w202) -> (.not. x?=w203:bool)
            n106 = Select(t=TypeDef_TDMS_States."Close" ("TDMS States"), s=w203, f=TypeDef_TDMS_States."Write" ("TDMS States")) -> (s? t:f=w201:T1)
          }
          frame "Close" {
            n107 = TDMS Close(8:w216, 11:w215) -> (0:w214:errorcluster)  [unwired: 1 out]
          }
        }
        n108 = local read "stop"() -> (w137:bool)
        n109 = Equal?(x=w139, y=TypeDef_TDMS_States."WaitingForCreate" ("TDMS States")) -> (x = y?=w142:bool)
        n110 = Equal?(x=w139, y=TypeDef_TDMS_States."Close" ("TDMS States")) -> (x = y?=w141:bool)
        n111 = Or(x=w142, y=w141) -> (x .or. y?=w140:bool)
        n112 = And(x=w140, y=w137) -> (x .and. y?=w138:bool)
        n113 = node-c288() -> ()  [unwired: 1 in, 1 out]
        "TDMS States" <- w136
      }
      n114 = node-c288(w126) -> ()  [unwired: 1 out]
      n115 = node-c288(w134) -> ()  [unwired: 1 out]
    }
    frame #5 {
      # "Motor Current Setpoint"
      # "Tacho"
      # "Encoder Motor Side"
      # "Close Everything"
      n116 = call <vilib>:"Stop.vi"("Encoder Ref In"=w402) -> ("Encoder Ref Out"=w403:T27)  [unwired: 9 in, 1 out]
      n117 = Build Array(0.0) -> (w397:dbl[])
      n118 = call <vilib>:"Close.vi"("Encoder Ref In"=w403) -> ()  [unwired: 10 in, 1 out]
      n119 = call <vilib>:"Write.vi"("Values"=w397, "AO Ref In"=w399) -> ("AO Ref Out"=w400:T19)  [unwired: 7 in, 1 out]
      n120 = call <vilib>:"Close.vi"("AI Ref In"=w401) -> ()  [unwired: 10 in, 1 out]
      n121 = call <vilib>:"Close.vi"("AO Ref In"=w404) -> ()  [unwired: 10 in, 1 out]
      n122 = call <vilib>:"Close.vi"("AO Ref In"=w400) -> ()  [unwired: 10 in, 1 out]
    }
  }
